vi "SupresorRebotes2.vi"() -> ()   [LabVIEW 2018]
panel:
  out "Iteraciones":i32
  out "CNormal":i32
  out "CSinRebote":i32
  out "Señal Sin Rebote":bool
  in  "Señal Nueva":bool=TRUE
  in  "stop":bool
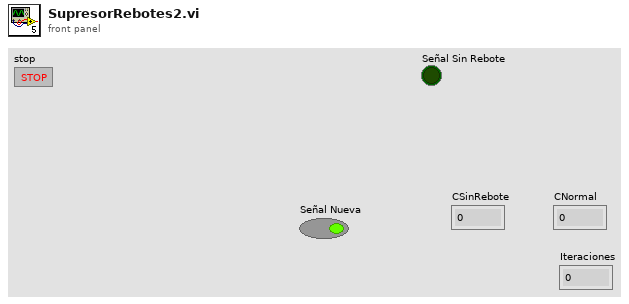
[diagram p1: front panel]
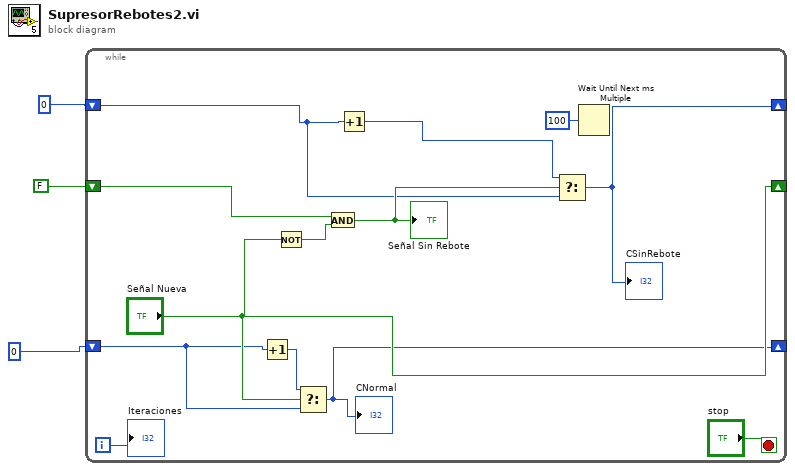
[diagram p0: block diagram]
diagram:
  n1 = while {
    shift-right: ["Señal Nueva"] -> _
    shift-left: FALSE -> [w14]
    shift-right: [w9] -> _
    shift-left: 0 -> [w10]
    shift-right: [w5] -> _
    shift-left: 0 -> [w6]
    i -> [w4]
    stop <- "stop" stop-if-true
    n2 = Increment(x=w6) -> (x+1=w7:i32)
    n3 = Not(x="Señal Nueva") -> (.not. x?=w13:bool)
    n4 = Select(t=w7, s="Señal Nueva", f=w6) -> (s? t:f=w5:i32)
    "CNormal" <- w5
    n5 = And(x=w14, y=w13) -> (x .and. y?=w12:bool)
    "Señal Sin Rebote" <- w12
    n6 = Increment(x=w10) -> (x+1=w11:i32)
    n7 = Select(t=w11, s=w12, f=w10) -> (s? t:f=w9:i32)
    "CSinRebote" <- w9
    n8 = Wait Until Next ms Multiple(millisecond multiple=u32 100) -> ()  [unwired: 1 out]
    "Iteraciones" <- w4
  }
